vi "18-Magnitude.vi"(11 "Snailfish Number in":string) -> (2 "Snailfish Number Magnitude":u64, 3 "Snailfish Number out":string)   [LabVIEW 2019, in "18.lvlib"]
uses:
  18.lvlib
  <vilib>/regexp/Match Regular Expression.xnode
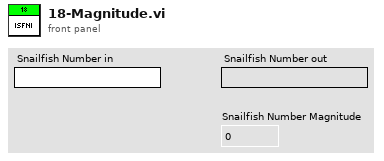
[diagram p1: front panel]
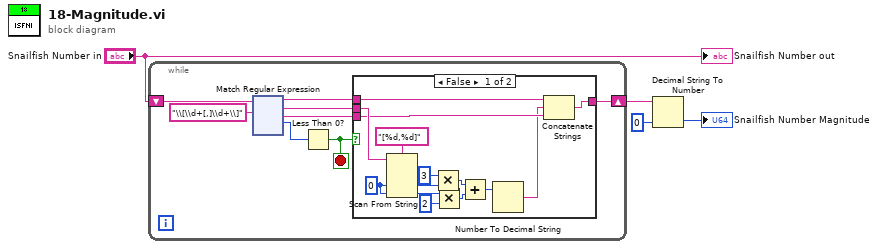
[diagram p0: block diagram]
diagram:
  n1 = while {
    shift-right: [w8] -> w3
    shift-left: "Snailfish Number in" -> [w12]
    stop <- w5 stop-if-true
    n2 = xnode "Match Regular Expression"("input string"=w12, "regular expression"="\\[\\d+[,]\\d+\\]") -> ("before match"=w10:string, "whole match"=w9:string, "after match"=w7:string, "offset past match"=w6:i32)  [unwired: 4 in, 1 out]
    n3 = Less Than 0?(x=w6) -> (x < 0?=w5:bool)
    n4 = case shown="False" w5 {
      tunnel: w10 -> [w26 w27]
      tunnel: w9 -> [w25 _]
      tunnel: [w16 w27] -> w8
      tunnel: w7 -> [w15 _]
      frame False {
        w21 = u64 0 ("default value 1")
        n5 = Scan From String(format string="[%d,%d]", input string=w25, default 1=w21, default 2=w21) -> (output 1=w23:u64, output 2=w20:u64)  [unwired: 2 in, 3 out]
        n6 = Multiply(x=u64 3, y=w23) -> (x*y=w18:u64)
        n7 = Multiply(x=w20, y=u64 2) -> (x*y=w17:u64)
        n8 = Add(x=w18, y=w17) -> (x+y=w14:u64)
        n9 = Number To Decimal String(number=w14) -> (decimal integer string=w13:string)  [unwired: 1 in]
        n10 = Concatenate Strings(w26, w13, w15) -> (w16:string)
      }
      frame True {
      }
    }
  }
  n11 = Decimal String To Number(string=w3, default (0L)=u64 0 ("default (0 I32)")) -> (number=→"Snailfish Number Magnitude":u64)  [unwired: 1 in, 1 out]
  "Snailfish Number out" <- "Snailfish Number in"
